vi "ProcessName.vi"() -> (1 "process name":string="CmsAcquisition")   [LabVIEW 2017, in "CmsAcquisition.lvlib"]
uses:
  <vilib>/addons/InsightCM/Devices/Shared/Cms/CmsAcquisition/CmsAcquisition.lvlib
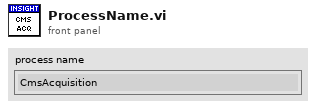
[diagram p1: front panel]
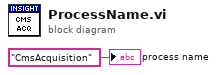
[diagram p0: block diagram]
diagram:
  "process name" <- "CmsAcquisition" ("ProcessName")
